vi "Vision Calculator.vi"(8 "Constants":T1, 10 "Corners":cluster{"Top Left":dbl[], "Bottom Right":dbl[]}, 11 "Gyro Heading":dbl) -> (0 "Angle to Target":dbl, 3 "Distance (ft)":dbl)   [LabVIEW 2015]
panel:
  out "Cam-field angle":dbl
  out "y_center":dbl
  out "x_center":dbl
  # "Local Variables"
  # "Inputs"
  # "Outputs"
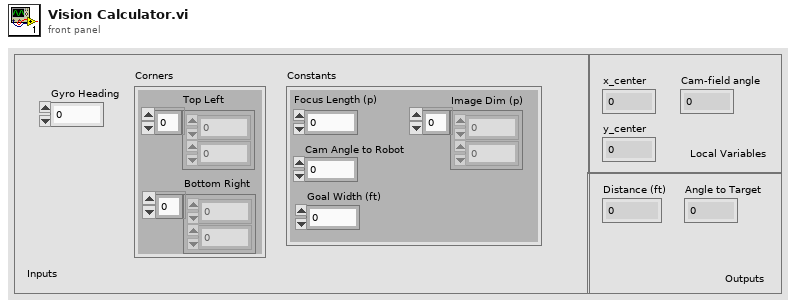
[diagram p1: front panel]
types:
  T1 = cluster{"Focus Length (p)":dbl, "Cam Angle to Robot":dbl, "Image Dim (p)":dbl[], "Goal Width (ft)":dbl}
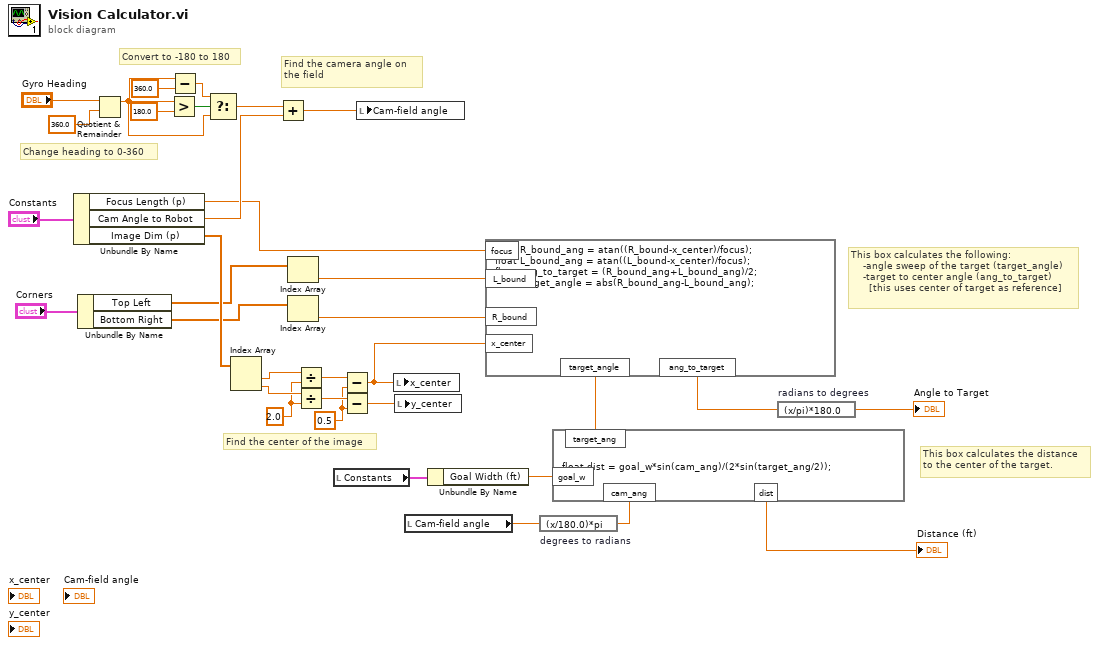
[diagram p0: block diagram]
diagram:
  w27 = 0.5 ("y")
  w30 = 2.0 ("y")
  # "This box calculates the distance\nto the center of the target."
  # "This box calculates the following:\n    -angle sweep of the target (target_angle)\n    -target to center angle (ang_to_target)\n      [this uses center of target as reference]"
  # "Find the camera angle on \nthe field"
  # "Convert to -180 to 180"
  # "Change heading to 0-360"
  # "Find the center of the image"
  n1 = Unbundle By Name("Constants") -> ("Focus Length (p)"=w10:dbl, "Cam Angle to Robot"=w17:dbl, "Image Dim (p)"=w33:dbl[])
  n2 = Unbundle By Name("Corners") -> ("Top Left"=w16:dbl[], "Bottom Right"=w15:dbl[])
  n3 = Quotient & Remainder(x="Gyro Heading", y=360.0) -> (x-y*floor(x/y)=w19:dbl)  [unwired: 1 out]
  n4 = Greater?(x=w19, y=180.0) -> (0:w23:bool)
  n5 = Subtract(x=w19, y=360.0) -> (x-y=w21:dbl)
  n6 = Select(t=w21, s=w23, f=w19) -> (s? t:f=w18:dbl)
  n7 = Index Array(array=w33) -> (element #1=w31:dbl, element #2=w32:dbl)  [unwired: 2 in]
  n8 = Add(x=w18, y=w17) -> (x+y=w8:dbl)
  n9 = Index Array(array=w16) -> (element=w14:dbl)  [unwired: 1 in]
  n10 = Index Array(array=w15) -> (element=w13:dbl)  [unwired: 1 in]
  n11 = Divide(x=w31, y=w30) -> (x/y=w29:dbl)
  n12 = Divide(x=w32, y=w30) -> (x/y=w28:dbl)
  n13 = local read "Constants"() -> (w9:T1)
  n14 = Subtract(x=w29, y=w27) -> (x-y=w12:dbl)
  n15 = Subtract(x=w28, y=w27) -> (x-y=w11:dbl)
  n16 = local write "Cam-field angle"(w8) -> ()
  n17 = local write "x_center"(w12) -> ()
  n18 = local write "y_center"(w11) -> ()
  n19 = local read "Cam-field angle"() -> (w2:dbl)
  n20 = Unbundle By Name(w9) -> ("Goal Width (ft)"=w7:dbl)
  n21 = formula code="float R_bound_ang = atan((R_bound-x_center)/focus);\nfloat L_bound_ang = atan((L_bound-x_center)/focus);\nfloat ang_to_target = (R_bound_ang+L_bound_ang)/2;\nfloat target_angle = abs(R_bound_ang-L_bound_ang);"("R_bound"=w13, "L_bound"=w14, "x_center"=w12, "focus"=w10) -> ("target_angle"=w6:dbl, "ang_to_target"=w3:dbl)
  n22 = expression code="(x/180.0)*pi" "degrees to radians"(w2) -> (w1:dbl)
  n23 = formula code="float dist = goal_w*sin(cam_ang)/(2*sin(target_ang/2));"("cam_ang"=w1, "goal_w"=w7, "target_ang"=w6) -> ("dist"=→"Distance (ft)":dbl)
  n24 = expression code="(x/pi)*180.0" "radians to degrees"(w3) -> (→"Angle to Target":dbl)
